vi "P-P Ripple.vi"(8 "error in":errorcluster, 9 "sampling time(S)":dbl=1.0 caption="min sample rate" format="%^.2e", 10 "Range":u16(ring) items=["0.2Vpp", "0.4Vpp", "1Vpp", "2Vpp", "4Vpp", "10Vpp", "20Vpp"], 11 "instrument handle":refnum<k15>) -> (0 "error out":errorcluster, 1 "wfm info":T1 {"reserved2" format="%.2f"; "reserved1" format="%.2f"; "offset" format="%^.3e"; "gain" format="%^.3e"; "xIncrement" format="%^.3e"; "relativeInitialX" format="%^.3e"; "absoluteInitialX" format="%^.3e"}, 2 "wfm":dbl[](array[numeric]), 3 "p-p Ripple":dbl)   [LabVIEW 2009]
doc: "NOTE: THIS FUNCTION WILL CLOBBER EXISTING DIGITIZER SETTINGS!!\n\nBe sure to restore all necessary digitizer configuration settings after using this VI."
uses:
  <instrlib>/niScope/Controls/niScope vertical coupling.ctl
  <instrlib>/niScope/Acquire/Fetch/niScope Fetch.vi
  <instrlib>/niScope/Configure/Trigger/niScope Configure Trigger Immediate.vi
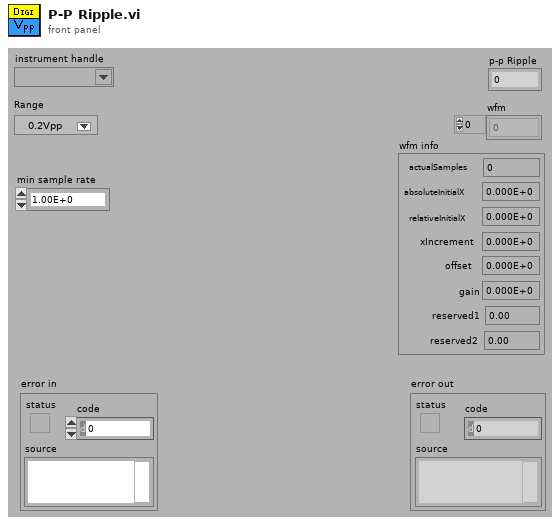
[diagram p1: front panel]
types:
  T1 = cluster{"actualSamples":i32, "absoluteInitialX":dbl, "relativeInitialX":dbl, "xIncrement":dbl, "offset":dbl, "gain":dbl, "reserved1":dbl, "reserved2":dbl}
  T2 = typedef "niScope vertical coupling.ctl" = i32
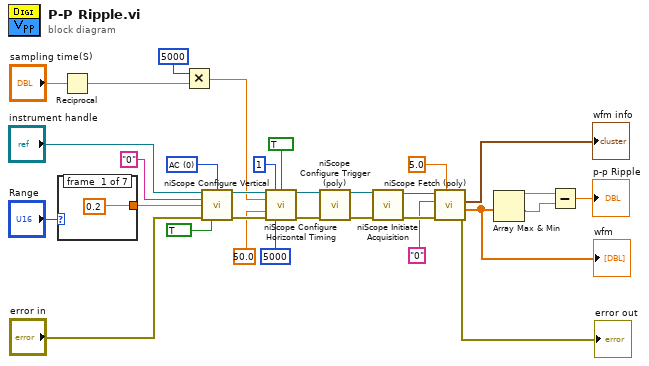
[diagram p0: block diagram]
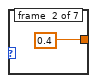
[diagram p2: hidden frame]
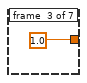
[diagram p3: hidden frame]
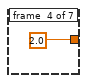
[diagram p4: hidden frame]
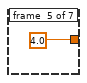
[diagram p5: hidden frame]
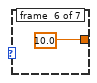
[diagram p6: hidden frame]
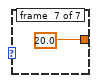
[diagram p7: hidden frame]
diagram:
  w29 = T2 0 items=["AC", "DC", "Ground"] ("vertical coupling")
  n1 = case shown="0, Default" "Range" {
    tunnel: [0.2 ("reference position") 0.4 ("reference position") 1.0 ("reference position") 2.0 ("reference position") 4.0 ("reference position") 10.0 ("reference position") 20.0 ("reference position")] -> w1
    frame #0 {
    }
    frame #1 {
    }
    frame #2 {
    }
    frame #3 {
    }
    frame #4 {
    }
    frame #5 {
    }
    frame #6 {
    }
  }
  n2 = Reciprocal(x="sampling time(S)") -> (1/x=w6:dbl)
  n3 = Multiply(x=5000 ("min record length"), y=w6) -> (x*y=w5:dbl)
  n4 = call <instrlib>:"niScope Configure Vertical.vi"("instrument handle"="instrument handle", "vertical coupling"=w29, "channels"="0", "vertical range"=w1, "error in"="error in", "channel enabled"=TRUE) -> ("instrument handle out"=w25:refnum<k15>, "error out"=w26:errorcluster)  [unwired: 8 in]
  n5 = call <instrlib>:"niScope Configure Horizontal Timing.vi"("instrument handle"=w25, "number of records"=1, "enforce realtime"=TRUE, "min sample rate"=w5, "reference position"=50.0, "error in"=w26, "min record length"=5000) -> ("instrument handle out"=w20:refnum<k15>, "error out"=w19:errorcluster)  [unwired: 7 in]
  n6 = call-poly <instrlib>:"niScope Configure Trigger (poly).vi"("instrument handle"=w20, "error in"=w19) -> ("instrument handle out"=w18:refnum<k15>, "error out"=w17:errorcluster)  [unwired: 12 in]
  n7 = call <instrlib>:"niScope Initiate Acquisition.vi"("instrument handle"=w18, "error in"=w17) -> ("instrument handle out"=w15:refnum<k15>, "error out"=w16:errorcluster)  [unwired: 12 in]
  n8 = call-poly <instrlib>:"niScope Fetch (poly).vi"("timeout"=5.0, "error in"=w16, "channels"="0", "instrument handle"=w15) -> ("error out"=→"error out":errorcluster, "wfm"=w12:dbl[], "wfm info"=→"wfm info":T1)  [unwired: 4 in, 1 out]
  "wfm" <- w12
  n9 = Array Max & Min(array=w12) -> (max value=w10:dbl, min value=w9:dbl)  [unwired: 2 out]
  n10 = Subtract(x=w10, y=w9) -> (x-y=→"p-p Ripple":dbl)
